vi "ParseXML.vi"() -> ()   [LabVIEW 2013]
uses:
  <vilib>/xml/Load XML File.vi
  <vilib>/xml/Close Reference(Node).vi
  <vilib>/xml/NI_XML.lvlib
  <resource>/objmgr/DOMUserDefRef.rc
panel:
  out "Has Child Nodes":bool
  in  "XPath expression":string="office:body"
  out "node text":string
  out "error out":errorcluster
  out "XML":string
  in  "path to XML document":path
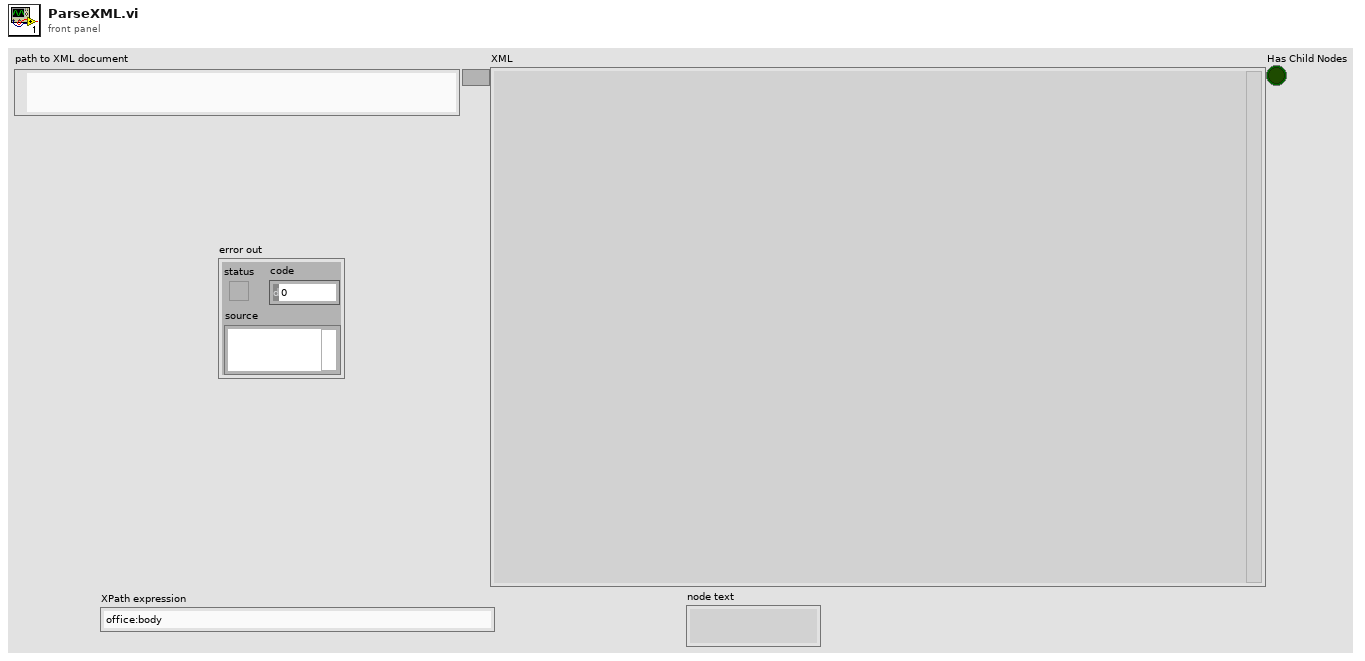
[diagram p1: front panel]
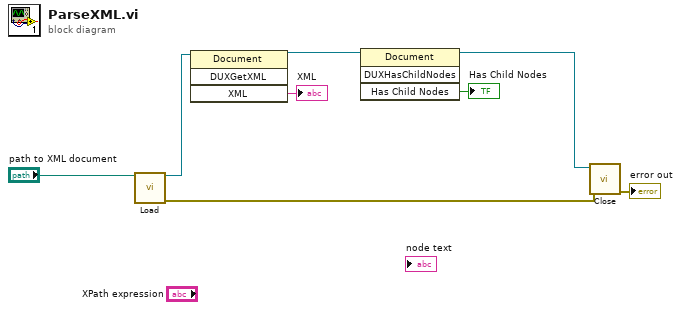
[diagram p0: block diagram]
diagram:
  n1 = call-poly <vilib>:"Load.vi"("path to XML document"="path to XML document") -> ("DOM document out"=w4:refnum<k20>, "error out"=w7:errorcluster)  [unwired: 12 in, 1 out]
  n2 = invoke class="Document" method="DUXGetXML"(reference=w4) -> (reference out=w3:refnum<k20>, "XML"=→"XML":string)  [unwired: 3 in, 2 out]
  n3 = invoke class="Document" method="DUXHasChildNodes"(reference=w3) -> (reference out=w1:refnum<k20>, "Has Child Nodes"=→"Has Child Nodes":bool)  [unwired: 3 in, 2 out]
  n4 = call-poly <vilib>:"Close.vi"("error in (no error)"=w7, "node"=w1) -> ("error out"=→"error out":errorcluster)  [unwired: 7 in]
